vi "Graph_Threshold_v00.vi"(6 "MaxMin":T1, 11 "Signals":T12={"PII In 1"={"Lock"=FALSE, "Hold"=FALSE, "P Gain"=0, "P BS"=0, "I Gain"=0, "I BS"=-10, "I2 G"=0, "I2 BS"=-26, "Scan Amp"=0, "Scan Off"=0, "Scan FS"=0, "SFS BS"=0, "I Max value"=10000, "I2 Max value"=10000, "Scope.Offset"=0, "Trigger Direction"=enum."either", "Scan-PII thresh"=0}, "PII In 2"={"Lock"=FALSE, "Hold"=FALSE, "P Gain"=0, "P BS"=0, "I Gain"=0, "I BS"=-10, "I2 G"=0, "I2 BS"=-26, "Scan Amp"=0, "Scan Off"=0, "Scan FS"=0, "SFS BS"=0, "I Max value"=10000, "I2 Max value"=10000, "Scope.Offset"=0, "Trigger Direction"=enum."either", "Scan-PII thresh"=0}, "PII In 3"={"Lock"=FALSE, "Hold"=FALSE, "P Gain"=0, "P BS"=0, "I Gain"=0, "I BS"=-10, "I2 G"=0, "I2 BS"=-26, "Scan Amp"=0, "Scan Off"=0, "Scan FS"=0, "SFS BS"=0, "I Max value"=10000, "I2 Max value"=10000, "Scope.Offset"=0, "Trigger Direction"=enum."either", "Scan-PII thresh"=0}, "PII In 4"={"Lock"=FALSE, "Hold"=FALSE, "P Gain"=0, "P BS"=0, "I Gain"=0, "I BS"=-10, "I2 G"=0, "I2 BS"=-26, "Scan Amp"=0, "Scan Off"=0, "Scan FS"=0, "SFS BS"=0, "I Max value"=10000, "I2 Max value"=10000, "Scope.Offset"=0, "Trigger Direction"=enum."either", "Scan-PII thresh"=0}, "PII In 5"={"Lock"=FALSE, "Hold"=FALSE, "P Gain"=0, "P BS"=-5, "I Gain"=0, "I BS"=-10, "I2 G"=0, "I2 BS"=-26, "Scan Amp"=0, "Scan Off"=0, "Scan FS"=0, "SFS BS"=0, "I Max value"=10000, "I2 Max value"=10000, "Scope.Offset"=0, "Trigger Direction"=enum."either", "Scan-PII thresh"=0}, "PII In 6"={"Lock"=FALSE, "Hold"=FALSE, "P Gain"=0, "P BS"=-10, "I Gain"=0, "I BS"=-10, "I2 G"=0, "I2 BS"=-26, "Scan Amp"=0, "Scan Off"=0, "Scan FS"=0, "SFS BS"=0, "I Max value"=10000, "I2 Max value"=10000, "Scope.Offset"=0, "Trigger Direction"=enum."either", "Scan-PII thresh"=0}, "Lock Thresh"={"Pump A"=2, "Pump B"=0, "EPR"=0, "Graph"=-10, "HD A"=0, "HD B"=-10}, "Re-Scan Thresh"={"Pump A"=2, "Pump B"=0, "EPR"=0, "Graph"=-10, "HD A"=0, "HD B"=-10}, "Safety First"={"lim reset"=FALSE, "no limit"=FALSE, "pos slew rate * dt"=10, "neg slew rate * dt"=-10, "Hold All"=FALSE, "Count(Ticks)"=0}, "Graph Errors"={"Pump A"=0, "Pump B"=1800, "EPR"=0, "Graph"=0, "HD A"=0, "HD B"=0}}) -> (3 "Control Graph Cluster":T8={"Control Pump A"={"Lock"=FALSE, "Hold"=FALSE, "P Gain"=0, "P BS"=-5, "I Gain"=0, "I BS"=-10, "I2 G"=0, "I2 BS"=-26, "Scan Amp"=0, "Scan Off"=0, "Scan FS"=0, "SFS BS"=0, "I Max value"=10000, "I2 Max value"=10000, "Scope.Offset"=0, "Trigger Direction"=enum."either", "Scan-PII thresh"=0}, "Control Pump B"={"Lock"=FALSE, "Hold"=FALSE, "P Gain"=0, "P BS"=-5, "I Gain"=0, "I BS"=-10, "I2 G"=0, "I2 BS"=-26, "Scan Amp"=0, "Scan Off"=0, "Scan FS"=0, "SFS BS"=0, "I Max value"=10000, "I2 Max value"=10000, "Scope.Offset"=0, "Trigger Direction"=enum."either", "Scan-PII thresh"=0}, "Control EPR"={"Lock"=FALSE, "Hold"=FALSE, "P Gain"=0, "P BS"=-5, "I Gain"=0, "I BS"=-10, "I2 G"=0, "I2 BS"=-26, "Scan Amp"=0, "Scan Off"=0, "Scan FS"=0, "SFS BS"=0, "I Max value"=10000, "I2 Max value"=10000, "Scope.Offset"=0, "Trigger Direction"=enum."either", "Scan-PII thresh"=0}, "Control Graph"={"Lock"=FALSE, "Hold"=FALSE, "P Gain"=0, "P BS"=-5, "I Gain"=0, "I BS"=-10, "I2 G"=0, "I2 BS"=-26, "Scan Amp"=0, "Scan Off"=0, "Scan FS"=0, "SFS BS"=0, "I Max value"=10000, "I2 Max value"=10000, "Scope.Offset"=0, "Trigger Direction"=enum."either", "Scan-PII thresh"=0}, "Control HD A"={"Lock"=FALSE, "Hold"=FALSE, "P Gain"=0, "P BS"=-5, "I Gain"=0, "I BS"=-10, "I2 G"=0, "I2 BS"=-26, "Scan Amp"=0, "Scan Off"=0, "Scan FS"=0, "SFS BS"=0, "I Max value"=10000, "I2 Max value"=10000, "Scope.Offset"=0, "Trigger Direction"=enum."either", "Scan-PII thresh"=0}, "Control HD B"={"Lock"=FALSE, "Hold"=FALSE, "P Gain"=0, "P BS"=-5, "I Gain"=0, "I BS"=-10, "I2 G"=0, "I2 BS"=-26, "Scan Amp"=0, "Scan Off"=0, "Scan FS"=0, "SFS BS"=0, "I Max value"=10000, "I2 Max value"=10000, "Scope.Offset"=0, "Trigger Direction"=enum."either", "Scan-PII thresh"=0}, "Max"={"Max Pump A"=0, "Max Pump B"=0, "Max EPR"=0, "Max Graph"=0, "Max HD A"=0, "Max HD B"=0}, "Min"={"Min Pump A"=0, "Min Pump B"=0, "Min EPR"=0, "Min Graph"=0, "Min HD A"=0, "Min HD B"=0}, "Lock Threshold"={"Pump A"=0, "Pump B"=0, "EPR"=0, "Graph"=0, "HD A"=0, "HD B"=0}, "Re-Scan Threshold"={"Pump A"=0, "Pump B"=0, "EPR"=0, "Graph"=0, "HD A"=40, "HD B"=0}, "Lock Point?"={"Pump A"=FALSE, "Pump B"=FALSE, "EPR"=FALSE, "Graph"=FALSE, "HD A"=FALSE, "HD B"=FALSE}, "Re-scan?"={"Pump A"=FALSE, "Pump B"=FALSE, "EPR"=FALSE, "Graph"=FALSE, "HD A"=FALSE, "HD B"=FALSE}, "Lock pressed? (-1)"={"Pump A"=FALSE, "Pump B"=FALSE, "EPR"=FALSE, "Graph"=FALSE, "HD A"=FALSE, "HD B"=FALSE}, "Cavity Errors"={"Pump A"=0, "Pump B"=0, "EPR"=0, "Graph"=0, "HD A"=0, "HD B"=0}, "State (-1)"={"Pump A"=enum."Safe", "Pump B"=enum."Safe", "EPR"=enum."Safe", "Graph"=enum."Safe", "HD A"=enum."Safe", "HD B"=enum."Safe"}, "Safety First"={"lim reset"=FALSE, "no limit"=FALSE, "pos slew rate * dt"=0, "neg slew rate * dt"=-5, "Hold All"=FALSE, "Count(Ticks)"=4294967286}})   [LabVIEW 2010]
doc: "Determines if the relative phase of the two interfering beams are within a range determined by a user-defined threshold. The absolute value of the error signal is used as a monitor."
uses:
  Strict Type Defs/Signals Graph.ctl
  Strict Type Defs/PII individual.ctl
  Strict Type Defs/Lock Thresh Graph.ctl
  Strict Type Defs/Safety First.ctl
  Strict Type Defs/Graph Errors.ctl
  Strict Type Defs/Graph Control Cluster.ctl
  Strict Type Defs/Graph Max.ctl
  Strict Type Defs/Graph Min.ctl
  Strict Type Defs/Graph Lock Point.ctl
  Strict Type Defs/Graph State.ctl
  Strict Type Defs/Graph MaxMin.ctl
  Strict Type Defs/Graph Reset MaxMin.ctl
panel:
  in  "Control Cavity Cluster":T8={"Control Pump A"={"Lock"=FALSE, "Hold"=FALSE, "P Gain"=0, "P BS"=-5, "I Gain"=0, "I BS"=-10, "I2 G"=0, "I2 BS"=-26, "Scan Amp"=0, "Scan Off"=0, "Scan FS"=0, "SFS BS"=0, "I Max value"=10000, "I2 Max value"=10000, "Scope.Offset"=0, "Trigger Direction"=enum."either", "Scan-PII thresh"=0}, "Control Pump B"={"Lock"=FALSE, "Hold"=FALSE, "P Gain"=0, "P BS"=-5, "I Gain"=0, "I BS"=-10, "I2 G"=0, "I2 BS"=-26, "Scan Amp"=0, "Scan Off"=0, "Scan FS"=0, "SFS BS"=0, "I Max value"=10000, "I2 Max value"=10000, "Scope.Offset"=0, "Trigger Direction"=enum."either", "Scan-PII thresh"=0}, "Control EPR"={"Lock"=FALSE, "Hold"=FALSE, "P Gain"=0, "P BS"=-5, "I Gain"=0, "I BS"=-10, "I2 G"=0, "I2 BS"=-26, "Scan Amp"=0, "Scan Off"=0, "Scan FS"=0, "SFS BS"=0, "I Max value"=10000, "I2 Max value"=10000, "Scope.Offset"=0, "Trigger Direction"=enum."either", "Scan-PII thresh"=0}, "Control Graph"={"Lock"=FALSE, "Hold"=FALSE, "P Gain"=0, "P BS"=-5, "I Gain"=0, "I BS"=-10, "I2 G"=0, "I2 BS"=-26, "Scan Amp"=0, "Scan Off"=0, "Scan FS"=0, "SFS BS"=0, "I Max value"=10000, "I2 Max value"=10000, "Scope.Offset"=0, "Trigger Direction"=enum."either", "Scan-PII thresh"=0}, "Control HD A"={"Lock"=FALSE, "Hold"=FALSE, "P Gain"=0, "P BS"=-5, "I Gain"=0, "I BS"=-10, "I2 G"=0, "I2 BS"=-26, "Scan Amp"=0, "Scan Off"=0, "Scan FS"=0, "SFS BS"=0, "I Max value"=10000, "I2 Max value"=10000, "Scope.Offset"=0, "Trigger Direction"=enum."either", "Scan-PII thresh"=0}, "Control HD B"={"Lock"=FALSE, "Hold"=FALSE, "P Gain"=0, "P BS"=-5, "I Gain"=0, "I BS"=-10, "I2 G"=0, "I2 BS"=-26, "Scan Amp"=0, "Scan Off"=0, "Scan FS"=0, "SFS BS"=0, "I Max value"=10000, "I2 Max value"=10000, "Scope.Offset"=0, "Trigger Direction"=enum."either", "Scan-PII thresh"=0}, "Max"={"Max Pump A"=0, "Max Pump B"=0, "Max EPR"=0, "Max Graph"=0, "Max HD A"=0, "Max HD B"=0}, "Min"={"Min Pump A"=0, "Min Pump B"=0, "Min EPR"=0, "Min Graph"=0, "Min HD A"=0, "Min HD B"=0}, "Lock Threshold"={"Pump A"=0, "Pump B"=0, "EPR"=0, "Graph"=0, "HD A"=0, "HD B"=0}, "Re-Scan Threshold"={"Pump A"=0, "Pump B"=0, "EPR"=0, "Graph"=0, "HD A"=40, "HD B"=0}, "Lock Point?"={"Pump A"=FALSE, "Pump B"=FALSE, "EPR"=FALSE, "Graph"=FALSE, "HD A"=FALSE, "HD B"=FALSE}, "Re-scan?"={"Pump A"=FALSE, "Pump B"=FALSE, "EPR"=FALSE, "Graph"=FALSE, "HD A"=FALSE, "HD B"=FALSE}, "Lock pressed? (-1)"={"Pump A"=FALSE, "Pump B"=FALSE, "EPR"=FALSE, "Graph"=FALSE, "HD A"=FALSE, "HD B"=FALSE}, "Cavity Errors"={"Pump A"=0, "Pump B"=0, "EPR"=0, "Graph"=0, "HD A"=0, "HD B"=0}, "State (-1)"={"Pump A"=enum."Safe", "Pump B"=enum."Safe", "EPR"=enum."Safe", "Graph"=enum."Safe", "HD A"=enum."Safe", "HD B"=enum."Safe"}, "Safety First"={"lim reset"=FALSE, "no limit"=FALSE, "pos slew rate * dt"=0, "neg slew rate * dt"=-5, "Hold All"=FALSE, "Count(Ticks)"=4294967286}}
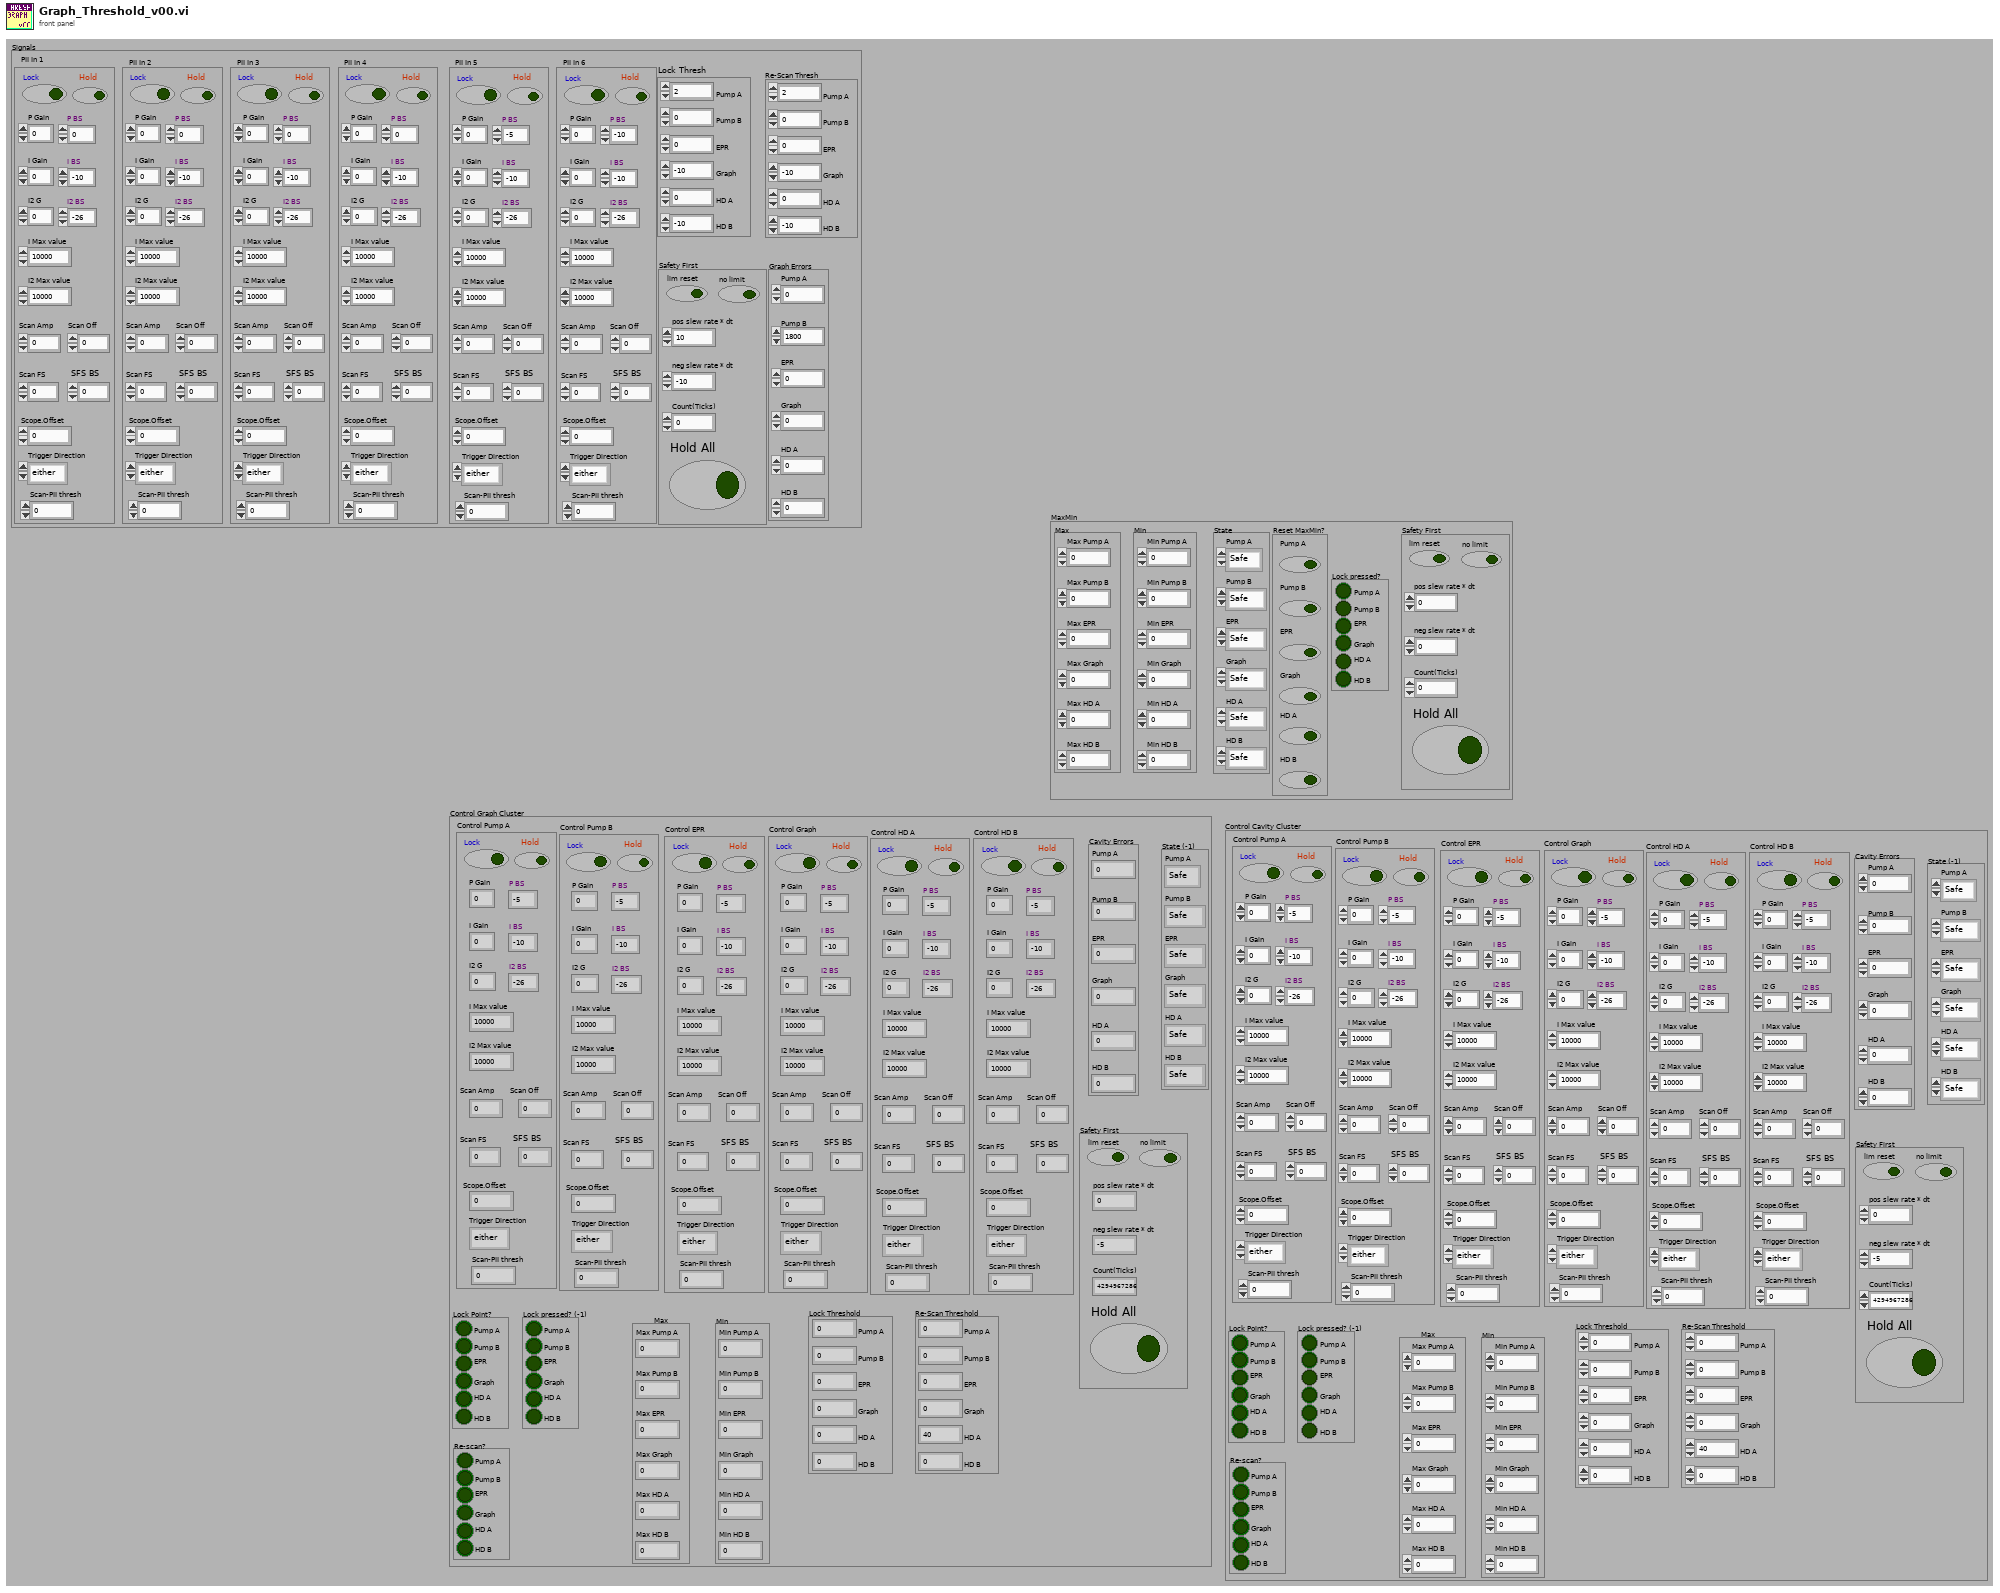
[diagram p1: front panel]
types:
  T1 = typedef "Graph MaxMin.ctl" = cluster{"State":T2, "Reset MaxMin?":T3, "Max":T4, "Min":T5, "Lock pressed?":T6, "Safety First":T7}
  T2 = typedef "Graph State.ctl" = cluster{"Pump A":enum16{"Safe", "Hold", "Scan", "Lock"}, "Pump B":enum16{"Safe", "Hold", "Scan", "Lock"}, "EPR":enum16{"Safe", "Hold", "Scan", "Lock"}, "Graph":enum16{"Safe", "Hold", "Scan", "Lock"}, "HD A":enum16{"Safe", "Hold", "Scan", "Lock"}, "HD B":enum16{"Safe", "Hold", "Scan", "Lock"}}
  T3 = typedef "Graph Reset MaxMin.ctl" = cluster{"Pump A":bool, "Pump B":bool, "EPR":bool, "Graph":bool, "HD A":bool, "HD B":bool}
  T4 = typedef "Graph Max.ctl" = cluster{"Max Pump A":i16, "Max Pump B":i16, "Max EPR":i16, "Max Graph":i16, "Max HD A":i16, "Max HD B":i16}
  T5 = typedef "Graph Min.ctl" = cluster{"Min Pump A":i16, "Min Pump B":i16, "Min EPR":i16, "Min Graph":i16, "Min HD A":i16, "Min HD B":i16}
  T6 = typedef "Graph Lock Point.ctl" = cluster{"Pump A":bool, "Pump B":bool, "EPR":bool, "Graph":bool, "HD A":bool, "HD B":bool}
  T7 = typedef "Safety First.ctl" = cluster{"lim reset":bool, "no limit":bool, "pos slew rate * dt":i16, "neg slew rate * dt":i16, "Hold All":bool, "Count(Ticks)":u32}
  T8 = typedef "Graph Control Cluster.ctl" = cluster{"Control Pump A":T9, "Control Pump B":T9, "Control EPR":T9, "Control Graph":T9, "Control HD A":T9, "Control HD B":T9, "Max":T4, "Min":T5, "Lock Threshold":T10, "Re-Scan Threshold":T10, "Lock Point?":T6, "Re-scan?":T6, "Lock pressed? (-1)":T6, "Cavity Errors":T11, "State (-1)":T2, "Safety First":T7}
  T9 = typedef "PII individual.ctl" = cluster{"Lock":bool, "Hold":bool, "P Gain":i32, "P BS":i16, "I Gain":i32, "I BS":i16, "I2 G":i32, "I2 BS":i16, "Scan Amp":i16, "Scan Off":i16, "Scan FS":u16, "SFS BS":i16, "I Max value":i32, "I2 Max value":i32, "Scope.Offset":i16, "Trigger Direction":enum8{"either", "minus-plus", "plus-minus"}, "Scan-PII thresh":i16}
  T10 = typedef "Lock Thresh Graph.ctl" = cluster{"Pump A":i16, "Pump B":i16, "EPR":i16, "Graph":i16, "HD A":i16, "HD B":i16}
  T11 = typedef "Graph Errors.ctl" = cluster{"Pump A":i16, "Pump B":i16, "EPR":i16, "Graph":i16, "HD A":i16, "HD B":i16}
  T12 = typedef "Signals Graph.ctl" = cluster{"PII In 1":T9, "PII In 2":T9, "PII In 3":T9, "PII In 4":T9, "PII In 5":T9, "PII In 6":T9, "Lock Thresh":T10, "Re-Scan Thresh":T10, "Safety First":T7, "Graph Errors":T11}
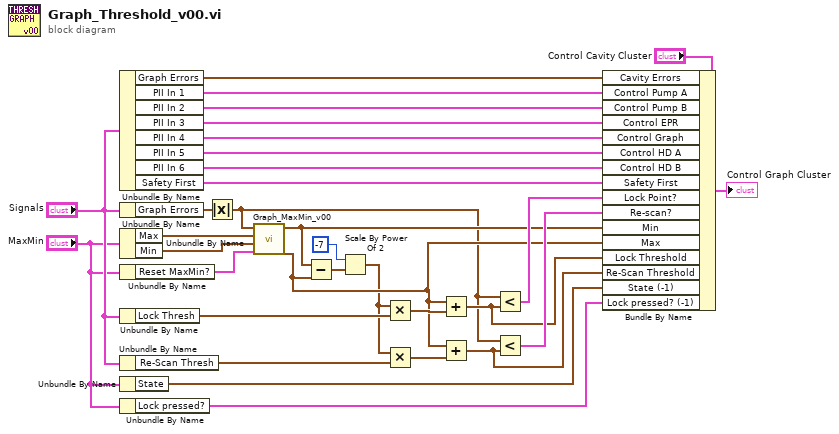
[diagram p0: block diagram]
diagram:
  n1 = Unbundle By Name("Signals") -> ("Graph Errors"=w19:T11, "PII In 1"=w18:T9, "PII In 2"=w17:T9, "PII In 3"=w16:T9, "PII In 4"=w15:T9, "PII In 5"=w6:T9, "PII In 6"=w5:T9, "Safety First"=w23:T7)
  n2 = Unbundle By Name("Signals") -> ("Graph Errors"=w4:T11)
  n3 = Unbundle By Name("MaxMin") -> ("Max"=w32:T4, "Min"=w31:T5)
  n4 = Unbundle By Name("MaxMin") -> ("Reset MaxMin?"=w14:T3)
  n5 = Unbundle By Name("Signals") -> ("Lock Thresh"=w2:T10)
  n6 = Unbundle By Name("Signals") -> ("Re-Scan Thresh"=w26:T10)
  n7 = Unbundle By Name("MaxMin") -> ("State"=w9:T2)
  n8 = Unbundle By Name("MaxMin") -> ("Lock pressed?"=w7:T6)
  n9 = Absolute Value(x=w4) -> (abs(x)=w3:T11)
  n10 = call "Graph_MaxMin_v00.vi"("Reset MaxMin?"=w14, "Min (-1)"=w31, "Max (-1)"=w32, "Graph Errors"=w3) -> ("Max"=w12:T4, "Min"=w13:T5)  [unwired: 6 in]
  n11 = Subtract(x=w13, y=w12) -> (x-y=w29:T5)
  n12 = Scale By Power Of 2(n=-7, x=w29) -> (x*2^n=w1:T5)
  n13 = Multiply(x=w1, y=w2) -> (x*y=w28:T5)
  n14 = Multiply(x=w1, y=w26) -> (x*y=w27:T5)
  n15 = Add(x=w12, y=w28) -> (x+y=w11:T4)
  n16 = Add(x=w12, y=w27) -> (x+y=w10:T4)
  n17 = Less?(x=w3, y=w11) -> (x < y?=w22:cluster{bool, bool, bool, bool, bool, bool})
  n18 = Less?(x=w3, y=w10) -> (x < y?=w21:cluster{bool, bool, bool, bool, bool, bool})
  n19 = Bundle By Name(cluster="Control Cavity Cluster", "Cavity Errors"=w19, "Control Pump A"=w18, "Control Pump B"=w17, "Control EPR"=w16, "Control Graph"=w15, "Control HD A"=w6, "Control HD B"=w5, "Safety First"=w23, "Lock Point?"=w22, "Re-scan?"=w21, "Min"=w13, "Max"=w12, "Lock Threshold"=w11, "Re-Scan Threshold"=w10, "State (-1)"=w9, "Lock pressed? (-1)"=w7) -> (→"Control Graph Cluster":T8)
